vi "find clumps.vi"(8 "error in (no error)":errorcluster, 11 "Channel Data In":T3[](array[typedef]) {"Mapping"."VS Reference" format="%.0x"}) -> (0 "error out":errorcluster, 2 "output accesses":T8[](array[typedef]) {"maps"."VS Reference" format="%.0x"}, 3 "input accesses":T1[](array[typedef]) {"Channel Data"."Mapping"."VS Reference" format="%.0x"})   [LabVIEW 2021]
uses:
  System Explorer/SubVIs/Modbus Type.ctl
  Shared/Modbus Master Shared.lvlib
  Shared/Controls/Data Model/DataType.ctl
  Shared/Controls/Data Model/Mapping.ctl
  Shared/Controls/Data Model/Channel.ctl
  Output Bulk Data Access.ctl
  Bulk Data Access.ctl
  <vilib>/NI VeriStand/Custom Device API/Custom Device Channel Type.ctl
  <vilib>/NI VeriStand/Custom Device API/Custom Device API.lvlib
  <vilib>/NI VeriStand/Custom Device API/Custom Device Item Ref.ctl
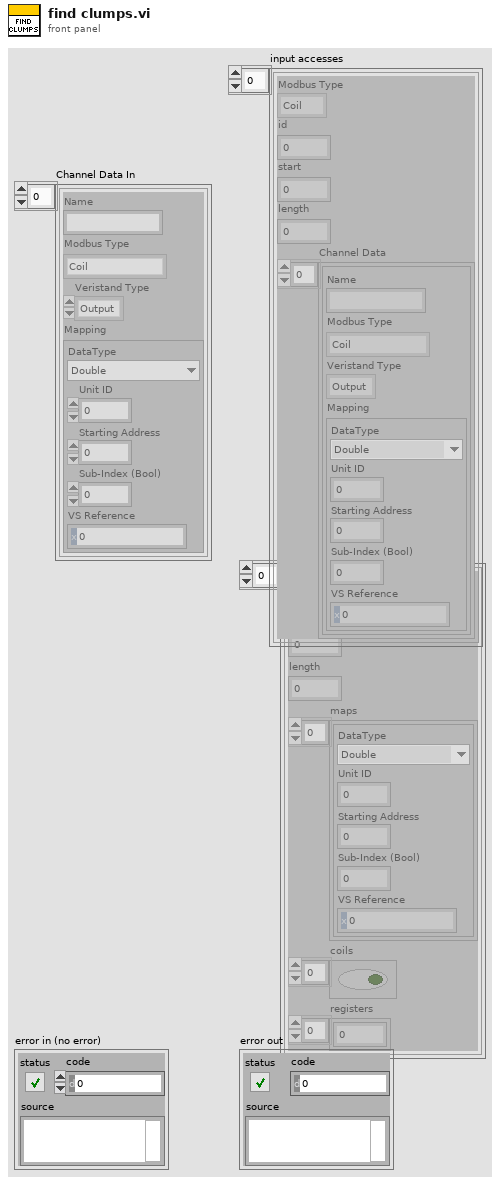
[diagram p1: front panel]
types:
  T1 = typedef "Modbus Master Shared.lvlib/Bulk Data Access.ctl" = cluster{"Modbus Type":T2, "id":u8, "start":u16, "length":u16, "Channel Data":T3[]}
  T2 = typedef "Modbus Master Shared.lvlib/Modbus Type.ctl" = enum16{"Coil", "Discrete Input", "Holding Register", "Input Register"}
  T3 = typedef "Modbus Master Shared.lvlib/Channel.ctl" = cluster{"Name":string, "Modbus Type":T2, "Veristand Type":T4, "Mapping":T5}
  T4 = typedef "Custom Device API.lvlib/Custom Device Channel Type.ctl" = enum16{"Input", "Output"}
  T5 = typedef "Modbus Master Shared.lvlib/Mapping.ctl" = cluster{"DataType":T6, "Unit ID":u8, "Starting Address":u16, "Sub-Index (Bool)":u16, "VS Reference":T7}
  T6 = typedef "Modbus Master Shared.lvlib/DataType.ctl" = enum16{"Double", "Single", "I64", "I32", "I16", "I8", "U64", "U32", "U16", "U8", "Boolean"}
  T7 = typedef "Custom Device API.lvlib/Custom Device Item Ref.ctl" = u64
  T8 = typedef "Modbus Master Shared.lvlib/Output Bulk Data Access.ctl" = cluster{"Modbus Type":T2, "start":u16, "length":u16, "maps":T5[], "coils":bool[], "registers":u16[]}
  T9 = typedef "Modbus Master Shared.lvlib/Clump Precursor.ctl" = cluster{"Modbus Type":T2, "Veristand Type":T4, "Channels":T10[]}
  T10 = typedef "Modbus Master Shared.lvlib/Channel.ctl" = cluster{"Name":string, "Modbus Type":T2, "Veristand Type":T4, "Mapping":T11}
  T11 = typedef "Modbus Master Shared.lvlib/Mapping.ctl" = cluster{"DataType":T6, "Starting Address":u16, "Sub-Index (Bool)":u16, "VS Reference":T7}
  T12 = typedef "Modbus Master Shared.lvlib/clump.ctl" = cluster{"Modbus Type":T2, "Veristand Type":T4, "start":i32, "length":i32, "channel indices":i32[]}
  T13 = typedef "Modbus Master Shared.lvlib/Output Bulk Data Access.ctl" = cluster{"Modbus Type":T2, "start":u16, "length":u16, "maps":T11[], "coils":bool[], "registers":u16[]}
  T14 = typedef "Modbus Master Shared.lvlib/Bulk Data Access.ctl" = cluster{"Modbus Type":T2, "start":u16, "length":u16, "Channel Data":T10[]}
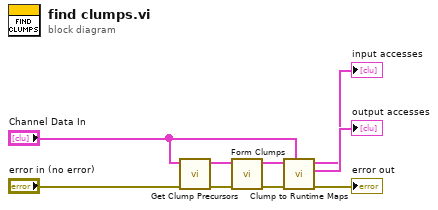
[diagram p0: block diagram]
diagram:
  n1 = call "Get Clump Precursors.vi"("error in (no error)"="error in (no error)", "Outputs.Channel Data.Coils"="Channel Data In") -> ("error out"=w3:errorcluster, "Clump Precursors"=w2:T9[])  [unwired: 8 in]
  n2 = call "Form Clumps.vi"("error in (no error)"=w3, "Clump Precursors"=w2) -> ("error out"=w9:errorcluster, "Clumps"=w8:T12[])  [unwired: 8 in]
  n3 = call "Clump to Runtime Maps.vi"("Channel Data"="Channel Data In", "error in (no error)"=w9, "Clumps"=w8) -> ("error out"=→"error out":errorcluster, "output accesses"=→"output accesses":T13[], "input accesses"=→"input accesses":T14[])  [unwired: 6 in]
